vi "Read Output Ch2.vi"(0 "VISA resource name":refnum<visa-resource-name>, 5 "Channel (1:Channel 1)":u16(ring)=1 items=["1"=1, "2"=2, "3"=3], 11 "error in (no error)":errorcluster) -> (4 "VISA resource name out":refnum<visa-resource-name>, 6 "Actual Voltage Level (V)":dbl format="%.4g", 8 "Actual Current Level (A)":dbl format="%.4g", 10 "Actual Power Level (W)":dbl format="%.4g", 15 "error out":errorcluster)   [LabVIEW 2017, in "BK Precision 913XX.lvlib"]
doc: "Returns the actual voltage, current, and power level of the output of the selected channel."
uses:
  <instrlib>/BK Precision 913XX/BK Precision 913XX.lvlib
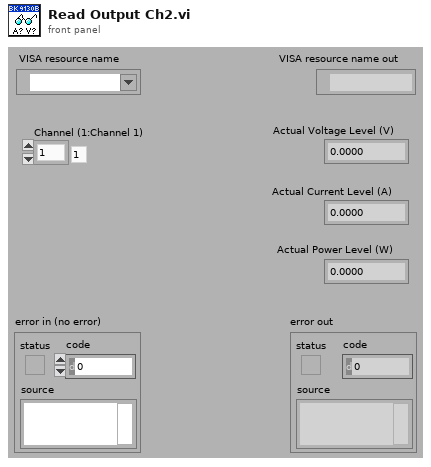
[diagram p1: front panel]
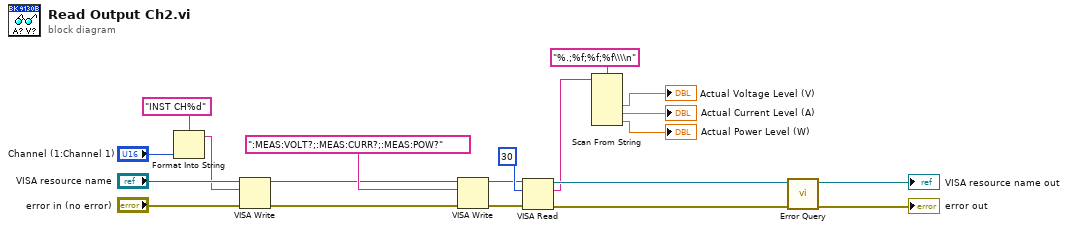
[diagram p0: block diagram]
diagram:
  n1 = Format Into String(format string="INST CH%d", "Channel (1:Channel 1)") -> (resulting string=w6:string)  [unwired: 2 in, 1 out]
  n2 = VISA Write(VISA resource name="VISA resource name", write buffer=w6, error in (no error)="error in (no error)") -> (VISA resource name out=w12:refnum<visa-resource-name>, error out=w11:errorcluster)  [unwired: 1 out]
  n3 = VISA Write(VISA resource name=w12, write buffer=":MEAS:VOLT?;:MEAS:CURR?;:MEAS:POW?", error in (no error)=w11) -> (VISA resource name out=w16:refnum<visa-resource-name>, error out=w15:errorcluster)  [unwired: 1 out]
  n4 = VISA Read(VISA resource name=w16, byte count=30, error in (no error)=w15) -> (VISA resource name out=w14:refnum<visa-resource-name>, read buffer=w5:string, error out=w13:errorcluster)  [unwired: 1 out]
  n5 = Scan From String(format string="%.;%f;%f;%f\\\\n", input string=w5) -> (output 1=→"Actual Voltage Level (V)":dbl, output 2=→"Actual Current Level (A)":dbl, output 3=→"Actual Power Level (W)":dbl)  [unwired: 5 in, 3 out]
  n6 = call <instrlib>:"Error Query.vi"("error in (no error)"=w13, "VISA resource name"=w14) -> ("error out"=→"error out":errorcluster, "VISA resource name out"=→"VISA resource name out":refnum<visa-resource-name>)  [unwired: 6 in, 2 out]
